vi "Ist mit Soll vergleichen UsrVal.vi"(8 "error in (no error)":errorcluster caption="Fehler (Eingang, kein Fehler)", 11 "Schneider Steuerung PNS Eingang":refnum<class "Schneider Steuerung PNS.lvclass">) -> (0 "error out":errorcluster caption="Fehler (Ausgang)", 2 "Werte":cluster{i32[], u16[]}, 3 "Schneider Steuerung PNS Ausgang":refnum<class "Schneider Steuerung PNS.lvclass">)   [LabVIEW 2020, in "Schneider Steuerung PNS.lvclass"]
uses:
  Schneider Steuerung PNS.lvclass
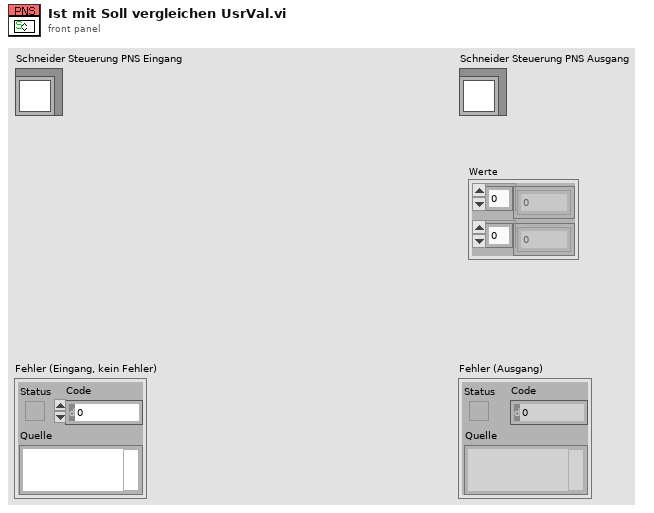
[diagram p1: front panel]
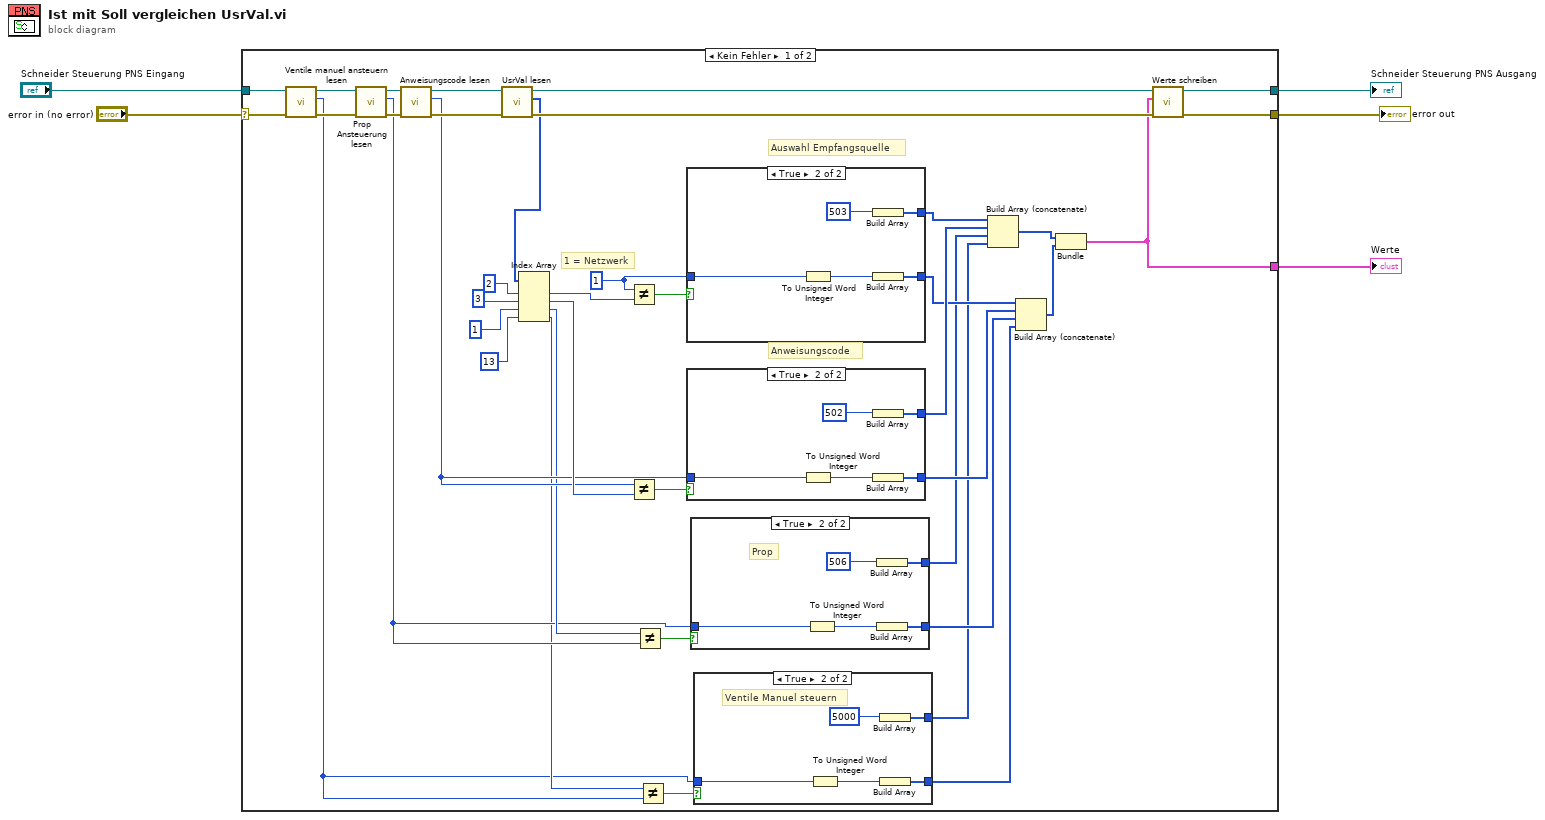
[diagram p0: block diagram]
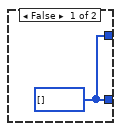
[diagram p2: hidden frame]
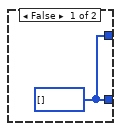
[diagram p3: hidden frame]
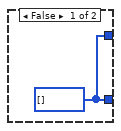
[diagram p4: hidden frame]
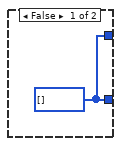
[diagram p5: hidden frame]
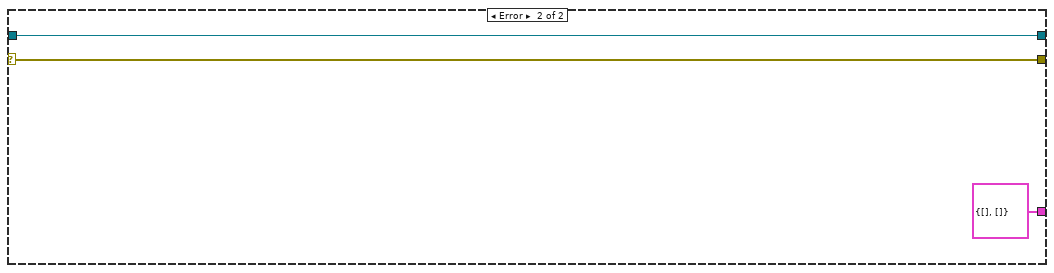
[diagram p6: hidden frame]
diagram:
  n1 = case shown="Kein Fehler" "error in (no error)" {
    selector: "error in (no error)" -> [w13 w72]
    tunnel: [w40 w72] -> w4
    tunnel: [w43 w71] -> w2
    tunnel: "Schneider Steuerung PNS Eingang" -> [w15 w71]
    tunnel: [w24 cluster{u16[], u16[]} {[], []}] -> w1
    frame No Error {
      w38 = u16 1 ("y")
      # "1 = Netzwerk"
      # "Anweisungscode"
      # "Auswahl Empfangsquelle"
      n2 = call-dynamic "Ventile manuel ansteuern lesen.vi"("error in (no error)"=w13, "Steuerung PNS (Eingang)"=w15) -> ("error out"=w12:errorcluster, "Ventile steuern"=w8:u16, "Steuerung PNS (Ausgang)"=w14:refnum<class "Schneider Steuerung PNS.lvclass">)  [unwired: 7 in]
      n3 = call-dynamic "Prop Ansteuerung lesen.vi"("error in (no error)"=w12, "Steuerung PNS (Eingang)"=w14) -> ("error out"=w21:errorcluster, "Propansteuerung"=w18:u16, "Steuerung PNS (Ausgang)"=w22:refnum<class "Schneider Steuerung PNS.lvclass">)  [unwired: 7 in]
      n4 = call-dynamic "Anweisungscode lesen.vi"("error in (no error)"=w21, "Steuerung PNS (Eingang)"=w22) -> ("error out"=w42:errorcluster, "Anweisungscode"=w28:u16, "Steuerung PNS (Ausgang)"=w45:refnum<class "Schneider Steuerung PNS.lvclass">)  [unwired: 7 in]
      n5 = call-dynamic "UsrVal lesen.vi"("error in (no error)"=w42, "Steuerung PNS (Eingang)"=w45) -> ("error out"=w41:errorcluster, "UsrVal"=w27:u16[], "Steuerung PNS (Ausgang)"=w44:refnum<class "Schneider Steuerung PNS.lvclass">)  [unwired: 7 in]
      n6 = Index Array(array=w27, index #1=2 ("Index"), index #2=3 ("Index"), index #3=1 ("Index"), index #4=13 ("Index")) -> (element #1=w37:u16, element #2=w34:u16, element #3=w20:u16, element #4=w10:u16)
      n7 = Not Equal?(x=w38, y=w37) -> (x != y?=w39:bool)
      n8 = Not Equal?(x=w28, y=w34) -> (x != y?=w36:bool)
      n9 = Not Equal?(x=w20, y=w18) -> (x != y?=w19:bool)
      n10 = Not Equal?(x=w10, y=w8) -> (x != y?=w11:bool)
      n11 = case shown="True" w39 {
        tunnel: w38 -> [_ w69]
        tunnel: [w64 w67] -> w33
        tunnel: [w64 w66] -> w31
        frame False {
          w64 = u16[] []
        }
        frame True {
          n12 = To Unsigned Word Integer(number=w69) -> (unsigned 16bit integer=w68:u16)
          n13 = Build Array(u16 503) -> (w67:u16[])
          n14 = Build Array(w68) -> (w66:u16[])
        }
      }
      n15 = case shown="True" w36 {
        tunnel: w28 -> [_ w63]
        tunnel: [w58 w61] -> w32
        tunnel: [w58 w60] -> w30
        frame False {
          w58 = u16[] []
        }
        frame True {
          n16 = To Unsigned Word Integer(number=w63) -> (unsigned 16bit integer=w62:u16)
          n17 = Build Array(u16 502) -> (w61:u16[])
          n18 = Build Array(w62) -> (w60:u16[])
        }
      }
      n19 = case shown="True" w19 {
        tunnel: w18 -> [_ w57]
        tunnel: [w52 w55] -> w17
        tunnel: [w52 w54] -> w16
        frame False {
          w52 = u16[] []
        }
        frame True {
          # "Prop"
          n20 = To Unsigned Word Integer(number=w57) -> (unsigned 16bit integer=w56:u16)
          n21 = Build Array(u16 506) -> (w55:u16[])
          n22 = Build Array(w56) -> (w54:u16[])
        }
      }
      n23 = case shown="True" w11 {
        tunnel: w8 -> [_ w51]
        tunnel: [w46 w49] -> w6
        tunnel: [w46 w48] -> w7
        frame False {
          w46 = u16[] []
        }
        frame True {
          # "Ventile Manuel steuern"
          n24 = To Unsigned Word Integer(number=w51) -> (unsigned 16bit integer=w50:u16)
          n25 = Build Array(u16 5000) -> (w49:u16[])
          n26 = Build Array(w50) -> (w48:u16[])
        }
      }
      n27 = Build Array (concatenate)(w33, w32, w17, w6) -> (w26:u16[])
      n28 = Build Array (concatenate)(w31, w30, w16, w7) -> (w25:u16[])
      n29 = Bundle(w26, w25) -> (w24:cluster{u16[], u16[]})  [unwired: 1 in]
      n30 = call-dynamic "Werte schreiben.vi"("error in (no error)"=w41, "Werte"=w24, "Steuerung PNS (Eingang)"=w44) -> ("error out"=w40:errorcluster, "Steuerung PNS (Ausgang)"=w43:refnum<class "Schneider Steuerung PNS.lvclass">)  [unwired: 7 in]
    }
    frame Error {
    }
  }
  "error out" <- w4
  "Schneider Steuerung PNS Ausgang" <- w2
  "Werte" <- w1
